vi "Set Color.vi"(8 "error in (no error)":errorcluster, 10 "Color (RGB black)":refnum<class "Color.lvclass">=refnum, 11 "Geometric Object.lvclass in":refnum<class "Graphics Object.lvclass">) -> (0 "error out":errorcluster, 3 "Geometric Object.lvclass out":refnum<class "Graphics Object.lvclass">)   [LabVIEW 2018, in "Graphics Object.lvclass"]
doc: "A method for setting the graphics object color"
uses:
  Graphics Object.lvclass
  Color/Color.lvclass
  RGB Color/RGB Color.lvclass
  Graphics Object.lvclass/Graphics Object.ctl
panel:
  # "expressionflow.com"
  # "Copyright (c) 2008 Tomi Maila. All rights reserved."
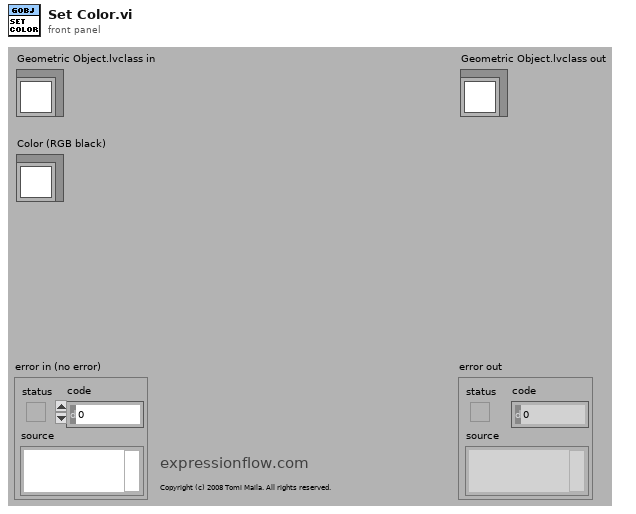
[diagram p1: front panel]
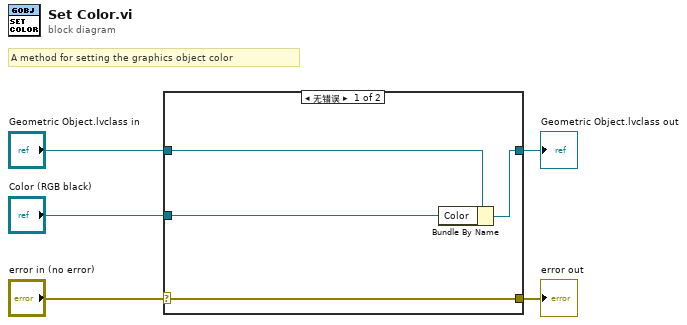
[diagram p0: block diagram]
diagram:
  # "A method for setting the graphics object color"
  n1 = case shown="无错误" "error in (no error)" {
    selector: "error in (no error)" -> [w9 w10]
    tunnel: [w9 w10] -> w4
    tunnel: [w7 w11] -> w2
    tunnel: "Geometric Object.lvclass in" -> [w8 w11]
    tunnel: "Color (RGB black)" -> [w6 _]
    frame No Error {
      n2 = Bundle By Name(cluster=w8, "Color"=w6) -> (w7:refnum<class "Graphics Object.lvclass">)
    }
    frame Error {
    }
  }
  "error out" <- w4
  "Geometric Object.lvclass out" <- w2
